vi "置反阈值.vi"(2 "Exit Event":refnum<user-event>) -> ()   [LabVIEW 2018]
uses:
  <vilib>/userdefined/High Color/IMAQdx.ctl
  <vilib>/vision/Image Controls.llb/IMAQ Image.ctl
  <vilib>/vision/driver/IMAQdx.llb/IMAQdx Acquisition Mode.ctl
  <vilib>/vision/NI_Vision_Development_Module.lvlib
  <vilib>/vision/driver/NI_Vision_Acquisition_Software.lvlib
panel:
  in  "Threshold Values":T1(slide)={"Minimum Value"=0.0, "Maximum Value"=99.65958} scale=0.0..255.0
  in  "Keep/Replace Value (Replace)":bool=TRUE
  in  "stop":bool
  in  "开始":bool
  in  "静态/实时":bool
  in  "Save Button":bool
  in  "IMAQdx Session":T2
  out "原图":T3(plugin-control)
  out "置反":T3(plugin-control)
  out "二值化":T3(plugin-control)
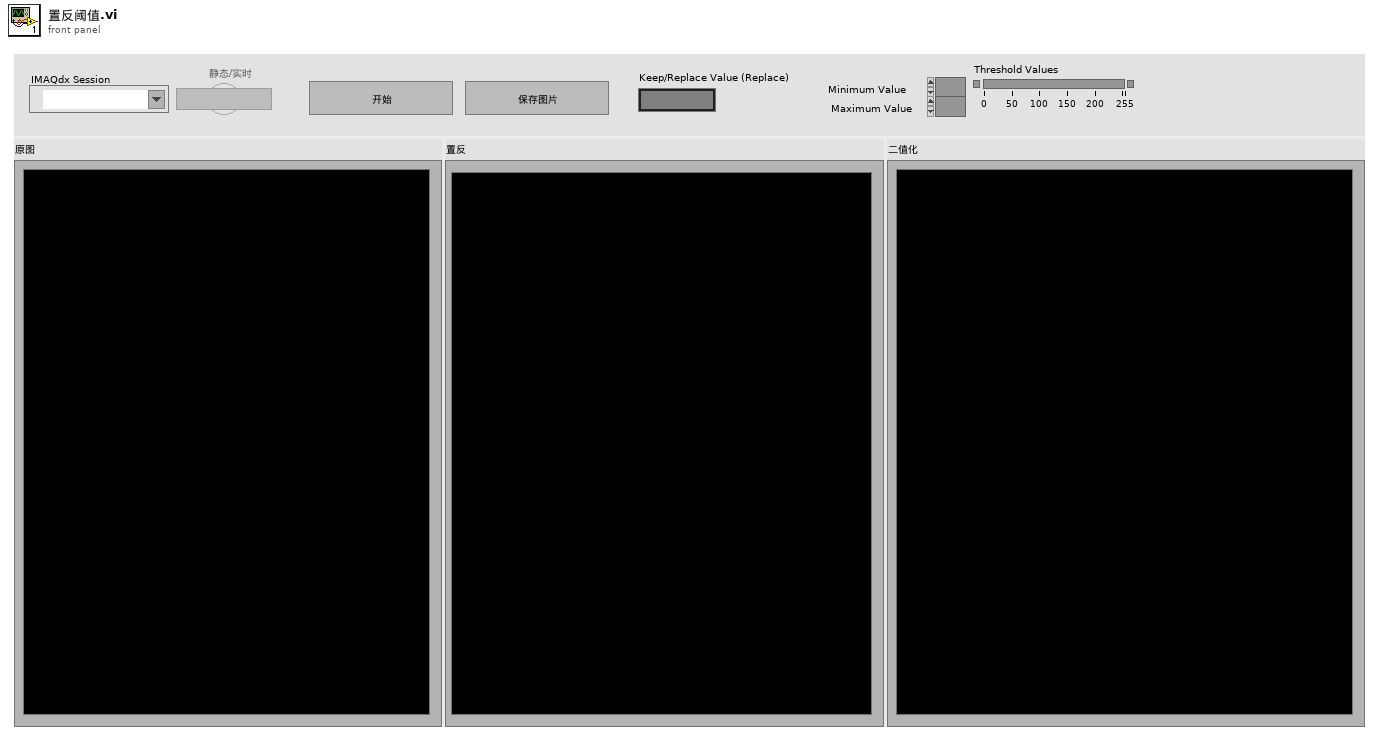
[diagram p1: front panel]
types:
  T1 = cluster{"Minimum Value":sgl, "Maximum Value":sgl}
  T2 = typedef "IMAQdx.ctl" = refnum<k21>
  T3 = typedef "IMAQ Image.ctl" = refnum<image>
  T4 = enum8{"Enabled", "Disabled", "Disabled and Grayed Out"}
  T5 = typedef "NI_Vision_Acquisition_Software.lvlib/IMAQdx Acquisition Mode.ctl" = enum32{"One Shot", "Continuous"}
  T6 = typedef "Image Type" = u32
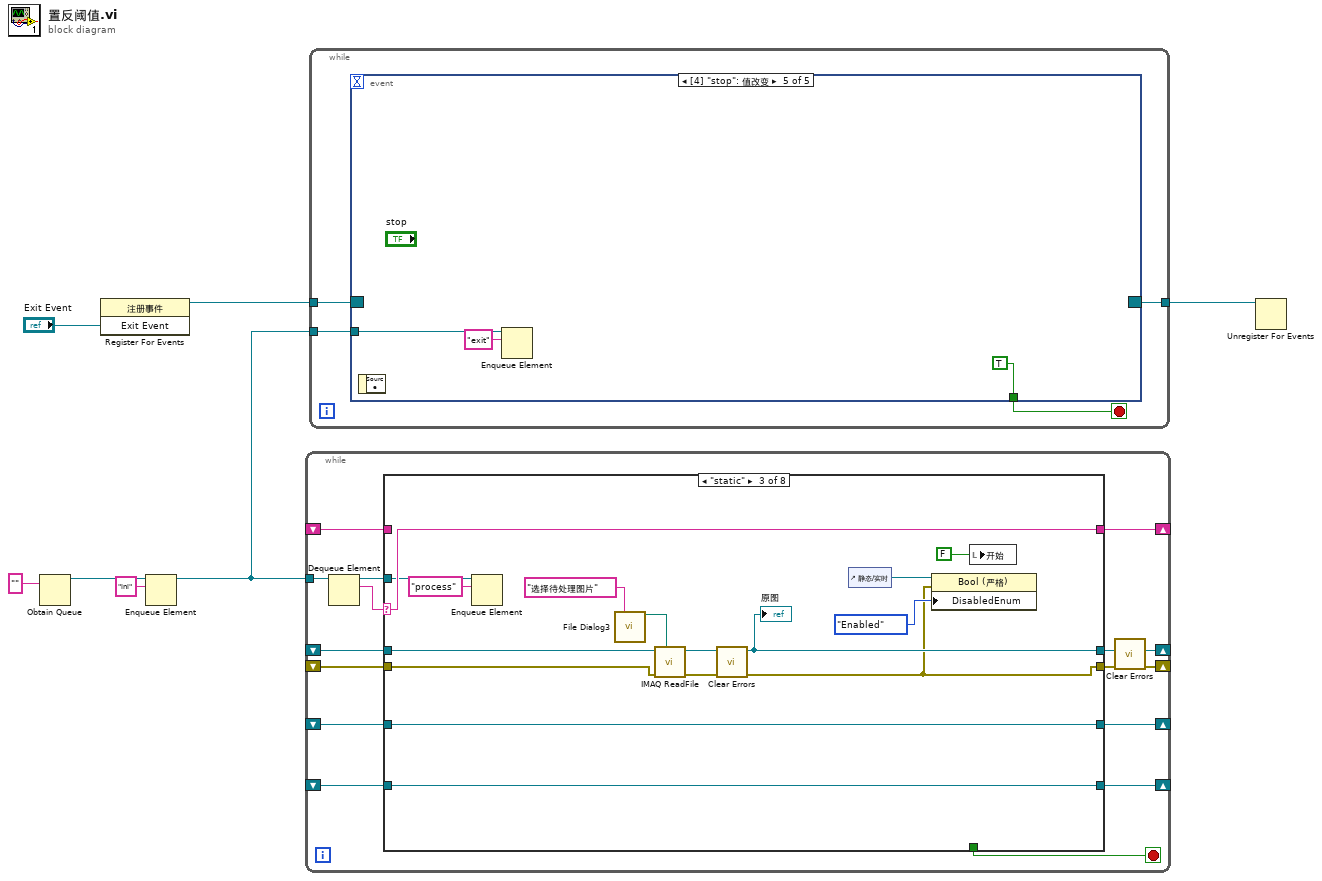
[diagram p0: block diagram]
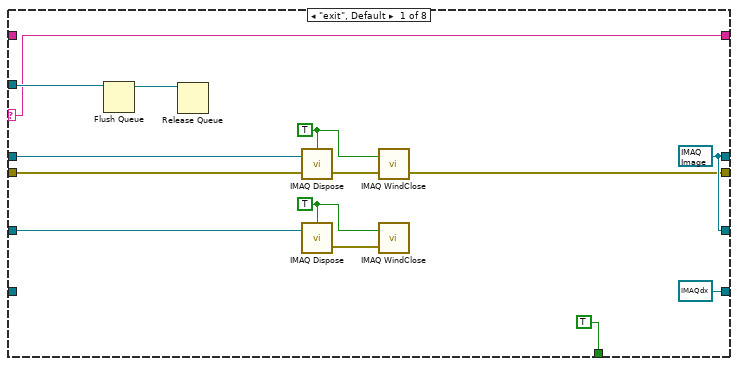
[diagram p2: hidden frame]
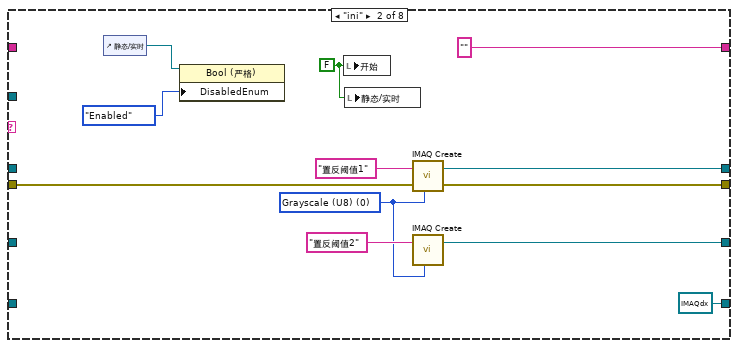
[diagram p3: hidden frame]
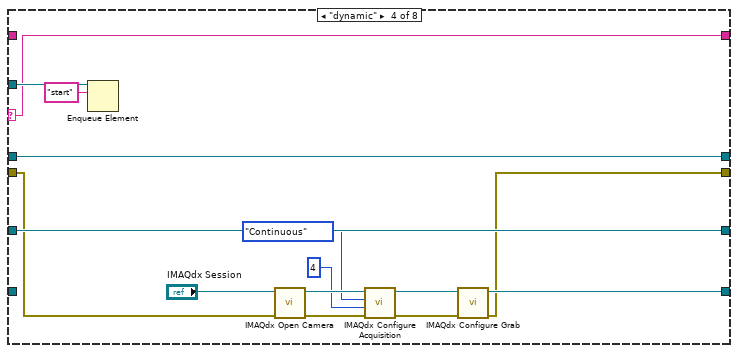
[diagram p4: hidden frame]
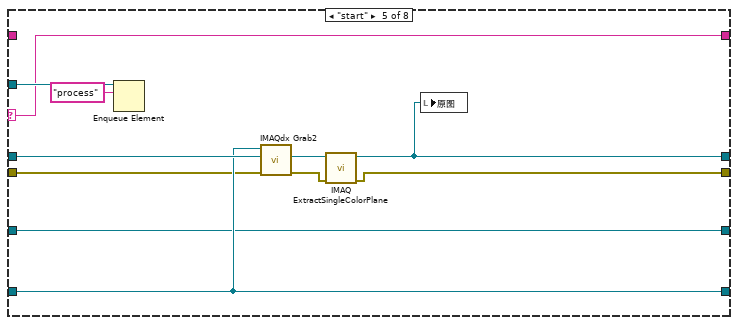
[diagram p5: hidden frame]
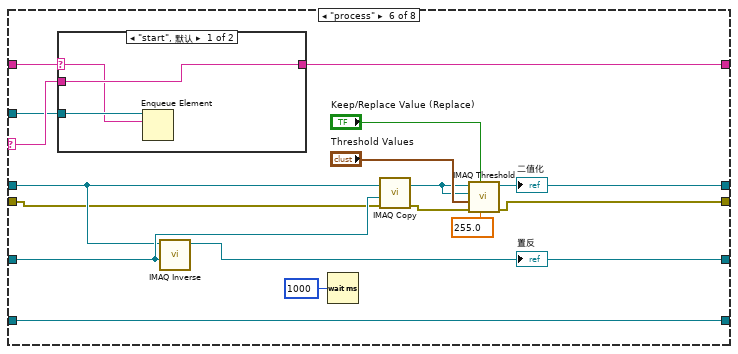
[diagram p6: hidden frame]
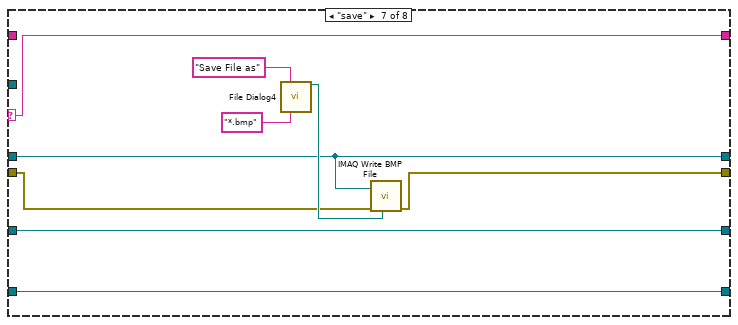
[diagram p8: hidden frame]
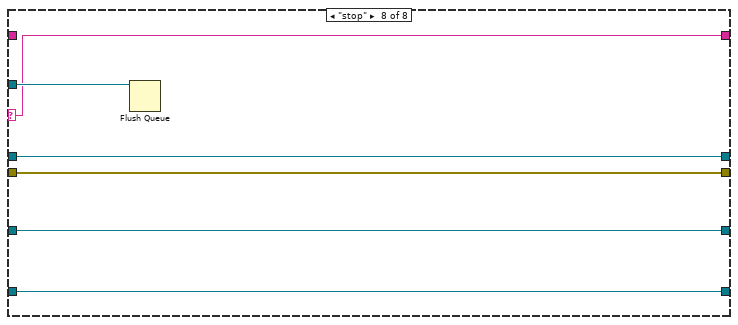
[diagram p9: hidden frame]
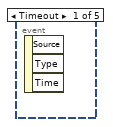
[diagram p10: hidden frame]
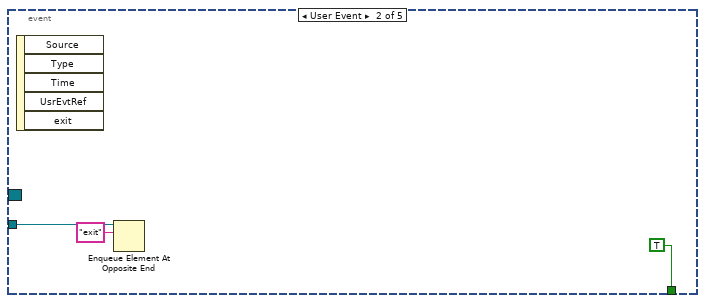
[diagram p11: hidden frame]
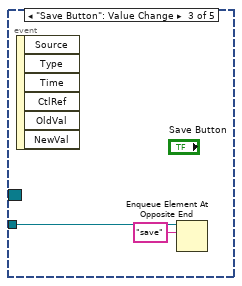
[diagram p12: hidden frame]
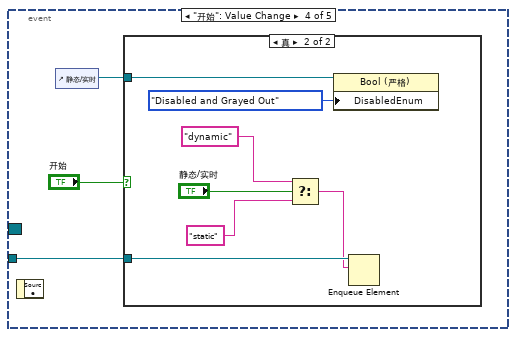
[diagram p13: hidden frame]
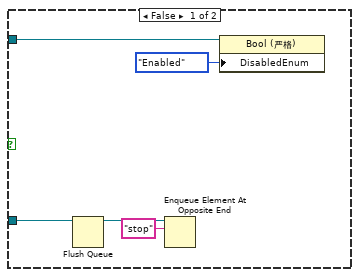
[diagram p14: hidden frame]
diagram:
  n1 = Obtain Queue(element data type="") -> (queue out=w4:refnum<queue>)  [unwired: 4 in, 2 out]
  n2 = register-events("Exit Event") -> (reference out=w1:refnum<event-registration>)  [unwired: 2 in, 1 out]
  n3 = Enqueue Element(queue=w4, element="ini") -> (queue out=w2:refnum<queue>)  [unwired: 2 in, 2 out]
  n4 = while {
    tunnel: w2 -> [w22]
    shift-right: [w18] -> _
    shift-left: _ -> [w17]
    shift-right: [w16] -> _
    shift-left: _ -> [w15]
    shift-right: [w14] -> _
    shift-left: _ -> [w13]
    shift-right: [w12] -> _
    shift-left: _ -> [w11]
    shift-right: [w8] -> _
    shift-left: _ -> [w9]
    stop <- w19 stop-if-true
    n5 = Dequeue Element(queue=w22) -> (queue out=w20:refnum<queue>, element=w21:string)  [unwired: 2 in, 2 out]
    n6 = case shown="\"static\"" w21 {
      selector: w21 -> [w29 _ w60 w75 w84 w104 w114 w122]
      tunnel: w20 -> [w36 _ w59 w77 w85 w102 _ w125]
      tunnel: [TRUE _ _ _ _ _ _ _] -> w19
      tunnel: [w28 w45 w52 w78 w87 w97 w116 w124] -> w18
      tunnel: w17 -> [w31 _ w56 w78 w88 w94 w116 w124]
      tunnel: [T2 refnum ("Session Out") T2 refnum ("Session Out") w61 w67 w86 w106 w115 w123] -> w16
      tunnel: w15 -> [_ _ w61 _ w86 w106 w115 w123]
      tunnel: [w29 "" w60 w75 w84 w103 w114 w122] -> w14
      tunnel: w13 -> [_ _ _ _ _ w105 _ _]
      tunnel: [w28 w39 w53 w74 w82 w101 w113 w121] -> w12
      tunnel: w11 -> [w25 _ w53 w74 w82 w96 w113 w121]
      tunnel: [w24 w38 w49 w64 w79 w91 w111 w120] -> w10
      tunnel: w9 -> [w23 w37 w50 w65 w81 w93 w112 w120]
      frame "exit", Default {
        w27 = TRUE ("All Images? (No)")
        w28 = T3 refnum ("New Image")
        w32 = TRUE ("All Images? (No)")
        n7 = Flush Queue(queue=w36) -> (queue out=w35:refnum<queue>)  [unwired: 1 in, 2 out]
        n8 = Release Queue(queue=w35) -> ()  [unwired: 2 in, 3 out]
        n9 = call "IMAQ Dispose"("All Images? (No)"=w32, "Image"=w31, "error in (no error)"=w23) -> ("error out"=w33:errorcluster)  [unwired: 3 in]
        n10 = call "IMAQ Dispose"("All Images? (No)"=w27, "Image"=w25) -> ("error out"=w26:errorcluster)  [unwired: 4 in]
        n11 = call "IMAQ WindClose"("Close All Windows (False)"=w32, "error in (no error)"=w33) -> ("error out"=w24:errorcluster)  [unwired: 4 in]
        n12 = call "IMAQ WindClose"("Close All Windows (False)"=w27, "error in (no error)"=w26) -> ()  [unwired: 4 in, 1 out]
      }
      frame "ini" {
        w42 = FALSE ("开始")
        w40 = T6 0 items=["Grayscale (U8)", "Grayscale (I16)", "Grayscale (SGL)", "Complex (CSG)", "RGB (U32)", "HSL (U32)", "RGB (U64)", "Grayscale (U16)"] ("Image Type")
        n13 = control-ref of="静态/实时"() -> (w44:refnum<vi>)
        n14 = property class="Bool (严格)"(reference=w44, "DisabledEnum"=T4."Enabled" ("Disabled")) -> ()  [unwired: 1 in, 2 out]
        n15 = local write "开始"(w42) -> ()
        n16 = local write "静态/实时"(w42) -> ()
        n17 = call "IMAQ Create"("Image Name"="置反阈值1", "Image Type"=w40, "error in (no error)"=w37) -> ("New Image"=w45:T3, "error out"=w38:errorcluster)  [unwired: 2 in]
        n18 = call "IMAQ Create"("Image Name"="置反阈值2", "Image Type"=w40) -> ("New Image"=w39:T3)  [unwired: 3 in, 1 out]
      }
      frame "static" {
        n19 = Enqueue Element(queue=w59, element="process") -> ()  [unwired: 2 in, 3 out]
        n20 = call "File Dialog3"("prompt"="选择待处理图片") -> ("selected path"=w63:path)  [unwired: 11 in, 3 out]
        n21 = call "IMAQ ReadFile"("File Path"=w63, "error in (no error)"=w50, "Image"=w56) -> ("error out"=w51:errorcluster, "Image Out"=w52:T3)  [unwired: 4 in, 3 out]
        "原图" <- w52
        n22 = call <vilib>:"Clear Errors.vi"("error in (no error)"=w51) -> ("error out"=w49:errorcluster)  [unwired: 5 in, 1 out]
        n23 = control-ref of="静态/实时"() -> (w55:refnum<vi>)
        n24 = property class="Bool (严格)"(reference=w55, error in=w49, "DisabledEnum"=T4."Enabled" ("Disabled")) -> ()  [unwired: 2 out]
        n25 = local write "开始"(FALSE ("开始")) -> ()
      }
      frame "dynamic" {
        n26 = Enqueue Element(queue=w77, element="start") -> ()  [unwired: 2 in, 3 out]
        n27 = call <vilib>:"IMAQdx Open Camera.vi"("error in"=w65, "Session In"="IMAQdx Session") -> ("error out"=w68:errorcluster, "Session Out"=w73:T2)  [unwired: 8 in]
        n28 = call <vilib>:"IMAQdx Configure Acquisition.vi"("error in"=w68, "Number of Buffers"=u32 4, "Continuous?"=IMAQdx_Acquisition_Mode."Continuous", "Session In"=w73) -> ("error out"=w69:errorcluster, "Session Out"=w70:T2)  [unwired: 6 in]
        n29 = call <vilib>:"IMAQdx Configure Grab.vi"("error in"=w69, "Session In"=w70) -> ("error out"=w64:errorcluster, "Session Out"=w67:T2)  [unwired: 8 in]
      }
      frame "start" {
        n30 = Enqueue Element(queue=w85, element="process") -> ()  [unwired: 2 in, 3 out]
        n31 = call <vilib>:"IMAQdx Grab2.vi"("error in"=w81, "Image In"=w88, "Session In"=w86) -> ("error out"=w80:errorcluster, "Image Out"=w89:T3)  [unwired: 5 in, 2 out]
        n32 = call "IMAQ ExtractSingleColorPlane"("error in (no error)"=w80, "Image Src"=w89) -> ("error out"=w79:errorcluster, "Image Dst Out"=w87:T3)  [unwired: 8 in]
        n33 = local write "原图"(w87) -> ()
      }
      frame "process" {
        n34 = case shown="\"start\", 默认" w105 {
          selector: w105 -> [w107 _]
          tunnel: w104 -> [w108 w110]
          tunnel: [w108 w110] -> w103
          tunnel: w102 -> [w109 _]
          frame "start", Default {
            n35 = Enqueue Element(queue=w109, element=w107) -> ()  [unwired: 2 in, 3 out]
          }
          frame "static" {
          }
        }
        n36 = call "IMAQ Inverse"("Image Dst"=w96, "Image Src"=w94) -> ("Image Dst Out"=w101:T3)  [unwired: 8 in, 1 out]
        "置反" <- w101
        n37 = Wait (ms)(milliseconds to wait=u32 1000 ("等待时间（毫秒）")) -> ()  [unwired: 1 out]
        n38 = call "IMAQ Copy"("error in (no error)"=w93, "Image Dst"=w96, "Image Src"=w94) -> ("error out"=w92:errorcluster, "Image Dst Out"=w95:T3)  [unwired: 3 in]
        n39 = call "IMAQ Threshold"("Replace Value"=sgl 255.0, "Keep/Replace Value (Replace)"="Keep/Replace Value (Replace)", "error in (no error)"=w92, "Range"="Threshold Values", "Image Dst"=w95, "Image Src"=w95) -> ("error out"=w91:errorcluster, "Image Dst Out"=w97:T3)  [unwired: 4 in]
        "二值化" <- w97
      }
      frame "save" {
        n40 = call "File Dialog4"("prompt"="Save File as", "pattern (all files)"="*.bmp" ("pattern")) -> ("selected path"=w119:path)  [unwired: 10 in, 3 out]
        n41 = call "IMAQ Write BMP File"("error in (no error)"=w112, "File Path"=w119, "Image"=w116) -> ("error out"=w111:errorcluster)  [unwired: 5 in]
      }
      frame "stop" {
        n42 = Flush Queue(queue=w125) -> ()  [unwired: 1 in, 3 out]
      }
    }
    n43 = call <vilib>:"Clear Errors.vi"("error in (no error)"=w10) -> ("error out"=w8:errorcluster)  [unwired: 5 in, 1 out]
  }
  n44 = while {
    tunnel: w1 -> [w129]
    tunnel: [w128] -> w6
    tunnel: w2 -> [w126]
    stop <- w127 stop-if-true
    n45 = event shown="[4] \"stop\": 值改变" {
      selector: w129 -> [_ _ _ _ _]
      dyn-events: [_ _ _ _ _] -> w128
      timeout: _ -> [_ _ _ _ _]
      tunnel: [_ TRUE _ _ TRUE] -> w127
      tunnel: w126 -> [_ w131 w134 w137 w151]
      event Timeout {
        n46 = event-data() -> ()  [unwired: 1 in, 3 out]
      }
      event User Event {
        n47 = event-data() -> ()  [unwired: 1 in, 5 out]
        n48 = Enqueue Element At Opposite End(queue=w131, element="exit") -> ()  [unwired: 2 in, 3 out]
      }
      event "Save Button": Value Change {
        n49 = event-data() -> ()  [unwired: 1 in, 6 out]
        n50 = Enqueue Element At Opposite End(queue=w134, element="save") -> ()  [unwired: 2 in, 3 out]
      }
      event "开始": Value Change {
        n51 = event-data() -> ()  [unwired: 1 in, 1 out]
        n52 = control-ref of="静态/实时"() -> (w135:refnum<vi>)
        n53 = case shown="真" "开始" {
          tunnel: w137 -> [w142 w149]
          tunnel: w135 -> [w138 w144]
          frame False {
            n54 = Flush Queue(queue=w142) -> (queue out=w141:refnum<queue>)  [unwired: 1 in, 2 out]
            n55 = Enqueue Element At Opposite End(queue=w141, element="stop") -> ()  [unwired: 2 in, 3 out]
            n56 = property class="Bool (严格)"(reference=w138, "DisabledEnum"=T4."Enabled" ("Disabled")) -> ()  [unwired: 1 in, 2 out]
          }
          frame True {
            n57 = Select(t="dynamic" ("f"), s="静态/实时", f="static" ("element")) -> (s? t:f=w147:string)
            n58 = property class="Bool (严格)"(reference=w144, "DisabledEnum"=T4."Disabled and Grayed Out" ("Disabled")) -> ()  [unwired: 1 in, 2 out]
            n59 = Enqueue Element(queue=w149, element=w147) -> ()  [unwired: 2 in, 3 out]
          }
        }
      }
      event "stop": Value Change {
        n60 = event-data() -> ()  [unwired: 1 in, 1 out]
        n61 = Enqueue Element(queue=w151, element="exit") -> ()  [unwired: 2 in, 3 out]
      }
    }
  }
  n62 = Unregister For Events(event registration refnum=w6) -> ()  [unwired: 1 in, 1 out]
